vi "Steer_PD_Control_Sim.vi"(6 "Steer_Angle":dbl, 7 "Steering Kd":dbl(slide)=0.9985221674876847 scale=0.1..2.0 scale format="%#_2g", 10 "Desired_Steer":dbl, 11 "Steering Kp":dbl) -> (2 "Vm":dbl)   [LabVIEW 2012]
uses:
  <vilib>/Simulation/Implementation/Shared/SIMSCR Execution Mode.ctl
  <vilib>/Simulation/Scripting/Companion Diagram/SimConfigNode/SimParams.ctl
  <vilib>/Simulation/Scripting/Companion Diagram/SimConfigNode/_simSolvers.ctl
  <vilib>/Simulation/Param Hierarchy/Typedefs/SIMPH Param Control Actions.ctl
  <vilib>/Simulation/Implementation/Shared/NILVSim_ParamChanged.vi
  <vilib>/Simulation/SignalArithmetic/Implementation/NILVSim Gain.llb/SIM Gain (scalar).vi
  <vilib>/Simulation/ContinuousLinear/Implementation/NILVSim Transfer Function Direct.llb/SIM Transfer Function Direct (SISO).vi
  <vilib>/Simulation/Nonlinear/Implementation/NILVSim Saturation.llb/SIM Saturation (scalar).vi
  <vilib>/Simulation/Implementation/Shared/NILVSim_Manager.vi
  <vilib>/Simulation/Implementation/Shared/NILVSim_FinalizeModel.vi
  <vilib>/Simulation/Implementation/Shared/SIM Unbundle Sim Info.vi
  <vilib>/Utility/error.llb/Clear Errors.vi
  <vilib>/Simulation/Implementation/Shared/NILVSim_GetModelError.vi
  <vilib>/Simulation/Implementation/Shared/SIM SimErrorHandler.vi
  <vilib>/Simulation/Implementation/Shared/SIM Bundle Sim Info.vi
  <vilib>/Simulation/Implementation/Shared/SIMSH Read Queue.vi
  <vilib>/Simulation/Implementation/Shared/NILVSim_Initialize.vi
  <vilib>/Simulation/Utility/Implementation/NILVSim Get Time and IsAcceptedStep.vi
  <vilib>/Simulation/Scripting/Companion Diagram/SimConfigNode/SimDog.xnode
  <vilib>/Simulation/Implementation/XNodeFramework/SimXNode/SimX.xnode
  <vilib>/Simulation/Implementation/Shared/NI_SIM_Implementation.lvlib
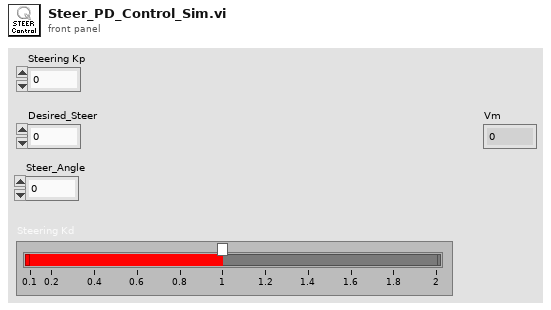
[diagram p1: front panel]
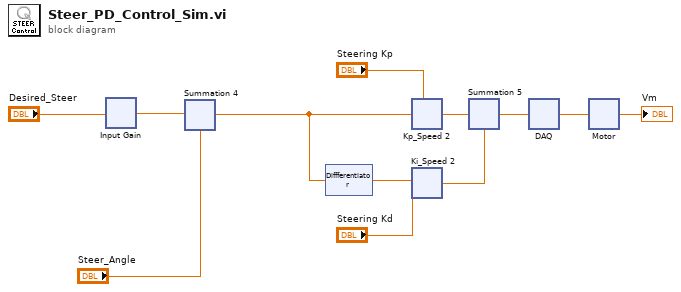
[diagram p0: block diagram]
diagram:
  n1 = xnode "Input Gain"("input"="Desired_Steer") -> ("output"=w1:dbl)  [unwired: 3 in]
  n2 = xnode ("Summation 4")("Operand1"=w1, "Operand2"="Steer_Angle") -> ("Result"=w10:dbl)
  n3 = xnode "Diffferentiator"("input u(k)"=w10) -> ("output y(k)"=w9:dbl)  [unwired: 4 in, 1 out]
  n4 = xnode ("Kp_Speed 2")("gain"="Steering Kp", "input"=w10) -> ("output"=w5:dbl)  [unwired: 2 in]
  n5 = xnode ("Ki_Speed 2")("gain"="Steering Kd", "input"=w9) -> ("output"=w6:dbl)  [unwired: 2 in]
  n6 = xnode ("Summation 5")("Operand1"=w5, "Operand2"=w6) -> ("Result"=w4:dbl)
  n7 = xnode "DAQ"("input"=w4) -> ("output"=w8:dbl)  [unwired: 4 in]
  n8 = xnode "Motor"("input"=w8) -> ("output"=→"Vm":dbl)  [unwired: 3 in]
